vi "thermal_optical_camera_V3.vi"() -> ()   [LabVIEW 2025]
panel:
  in  "File Path":string="C:\\Digambar\\Metal_thin_wall\\Optical_images\\Optical_images"
  in  "Stop (F)":bool
  in  "Acquisition Control:\nExposure Time [100, 3E7]":dbl=999.0 caption="Acquisition Control::Exposure Time" min=100.0 max=29999995.0
  in  "Analog Control:\nGain [0, 27]":dbl caption="Analog Control::Gain" min=0.0 max=27.045663671679687
  in  "Analog Control:\nBlack Level [-5, 10]":dbl caption="Analog Control::Black Level" min=-5.0000011920928955 max=10.000002384185791
  in  "Analog Control:\nGamma [0.25, 4.00]":dbl=0.800048828125 caption="Analog Control::Gamma" min=0.25 max=4.0 step=0.05
  out "Optical camera":T1(plugin-control)
  in  "optical capture interval (s)":dbl
  in  "thermal capture interval (s)":dbl
  out "Thermal camera":T1(plugin-control)
  out "IP address":string
  out "Output":string
  in  "Flag":bool
  in  "Stop recording":bool
  in  "Stop Preview":bool
  in  "Focus":dbl(slide) scale=0.0..100.0
  in  "Record":bool
  out "?":string
  # "Destination for Optical Images:"
  # "change folder name every time you run,\nso it saves each data set in dedicated folder:\nfolder1\nfolder2\nfolder3\netc..."
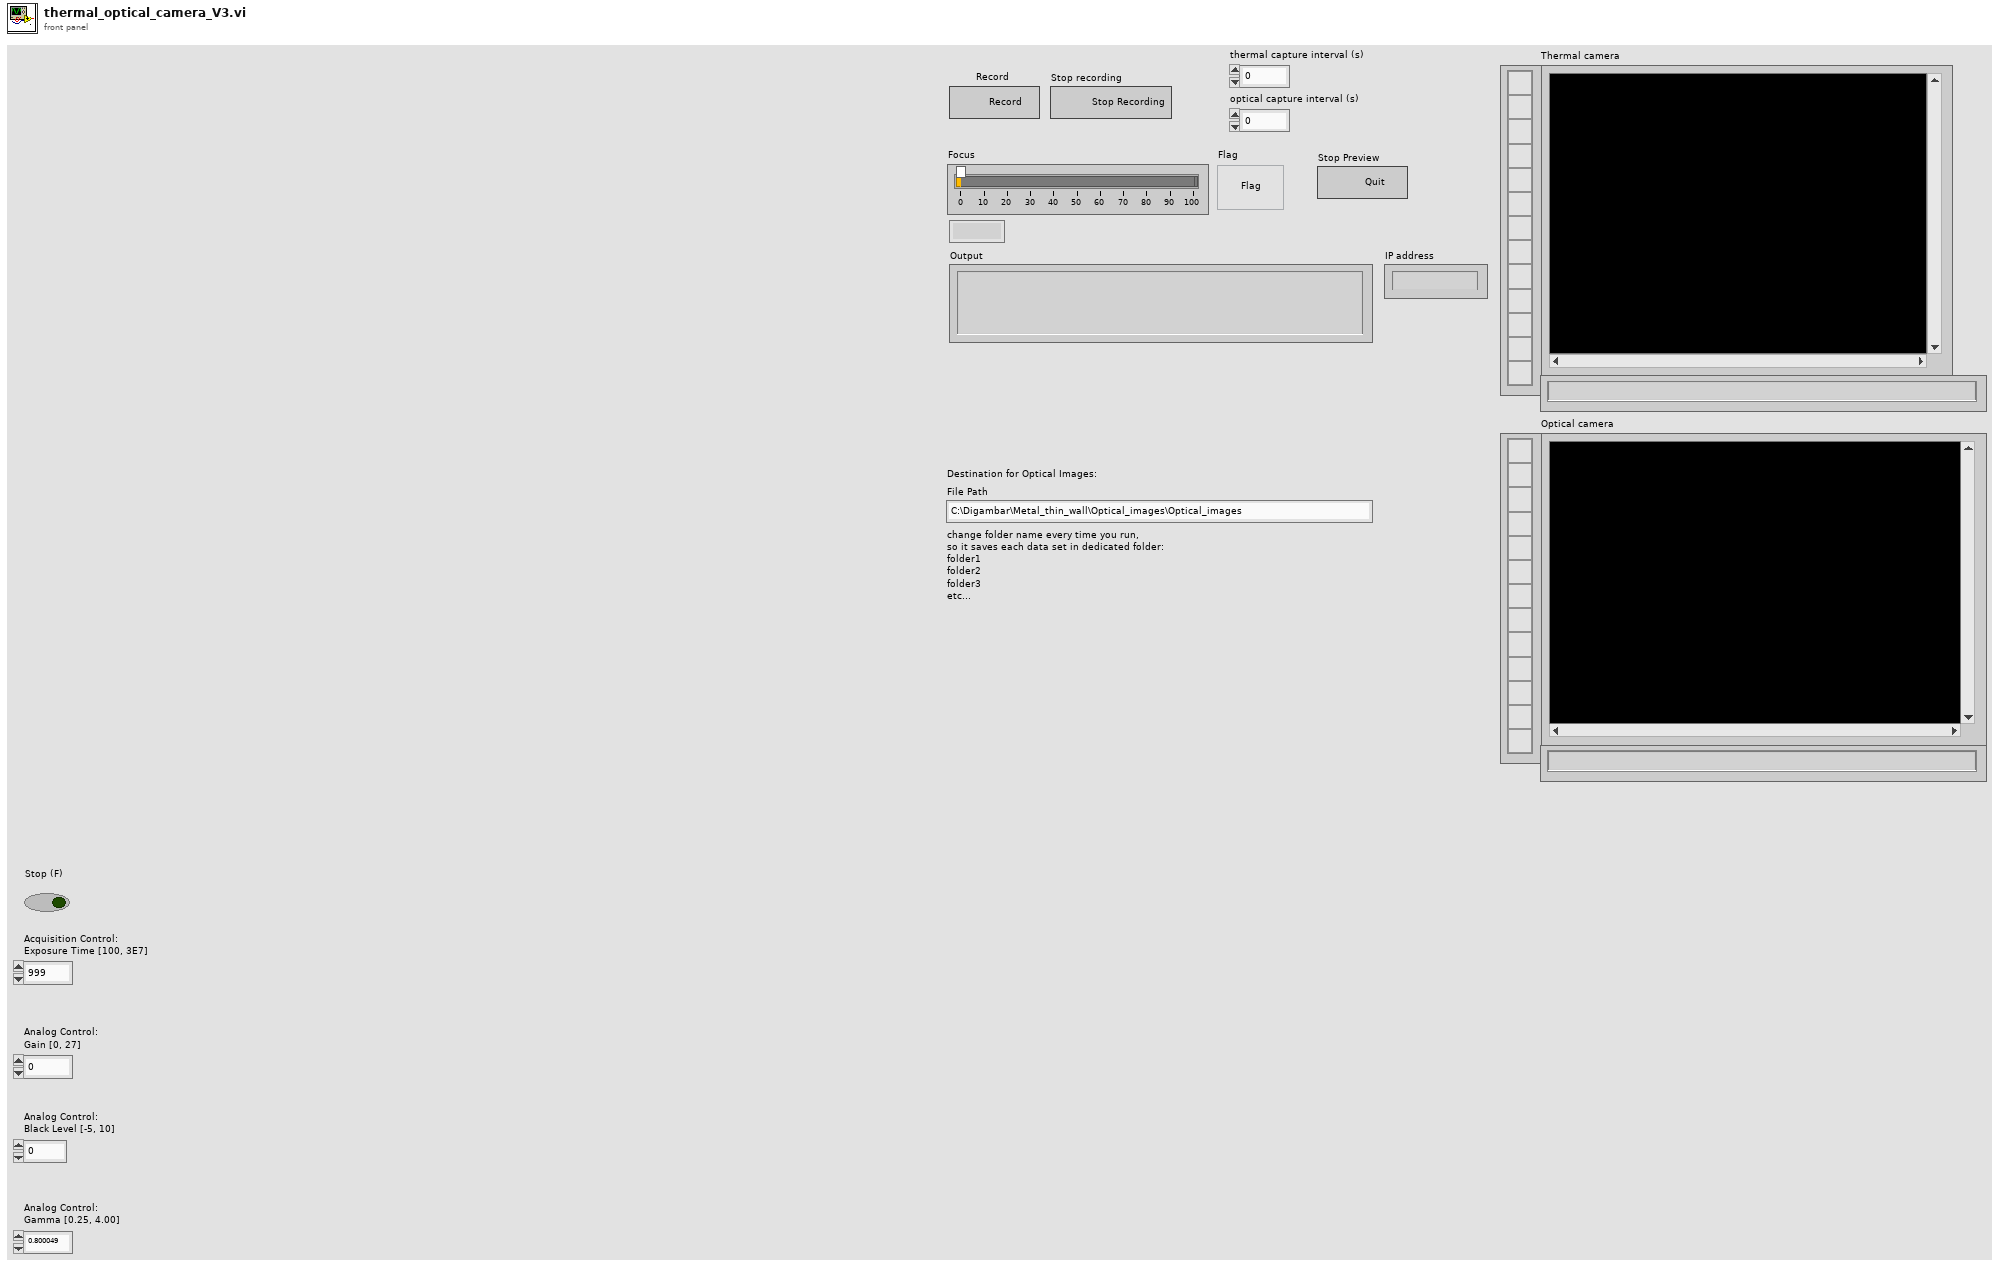
[diagram p1: front panel]
types:
  T1 = typedef "IMAQ Image.ctl" = refnum<image>
  T2 = enum16{"open", "replace", "create", "open or create", "replace or create", "replace or create with confirmation"}
  T3 = enum16{"big-endian, network order", "native, host order", "little-endian"}
  T4 = enum16{"Standard", "Buffered", "CRLF", "Immediate"}
  T5 = typedef "Image Type" = u32
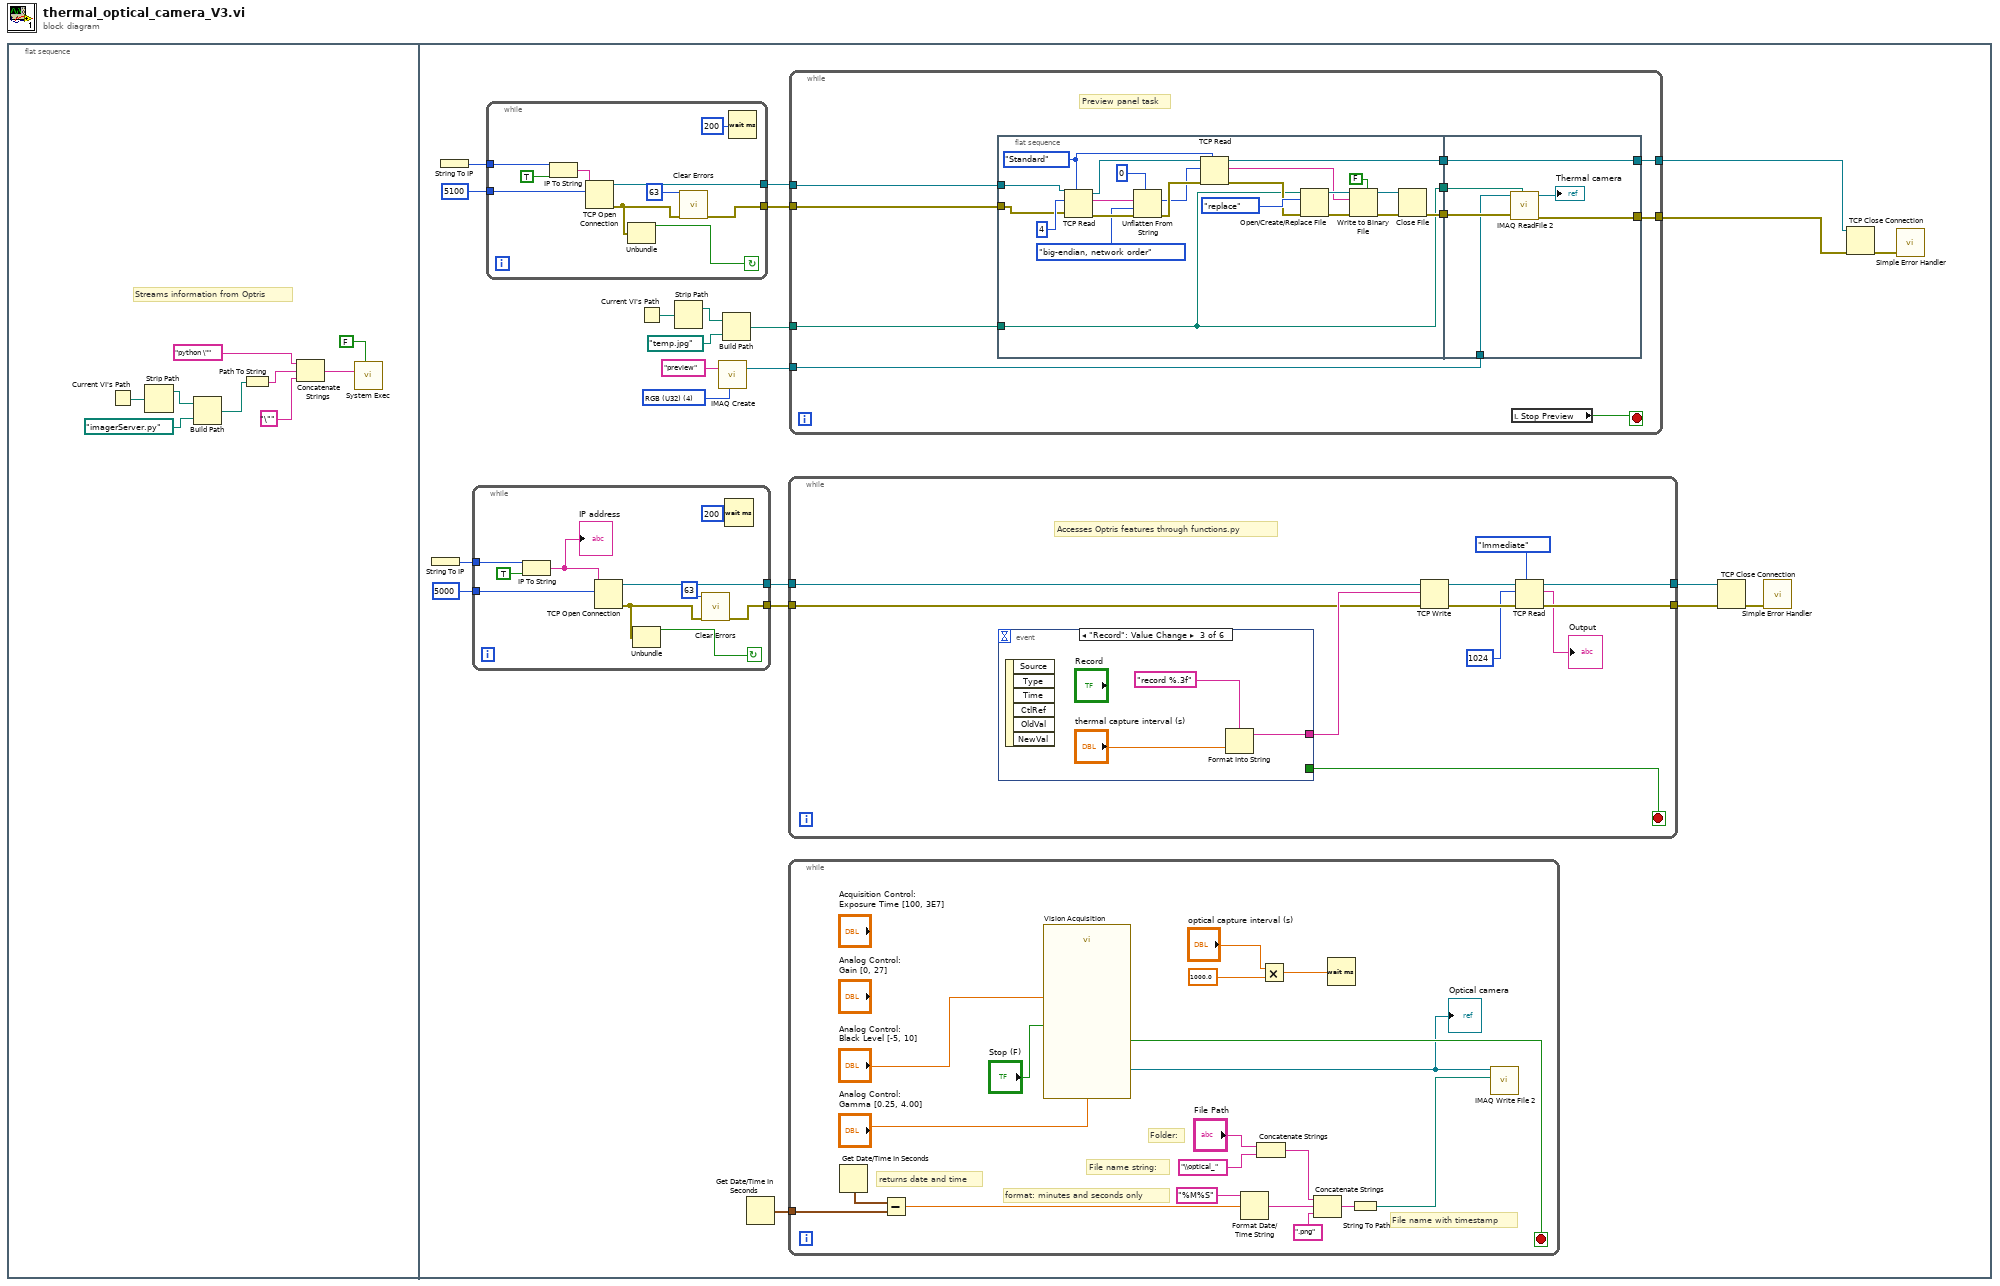
[diagram p0: block diagram]
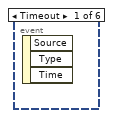
[diagram p2: hidden frame]
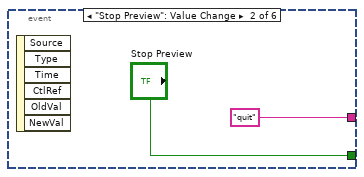
[diagram p3: hidden frame]
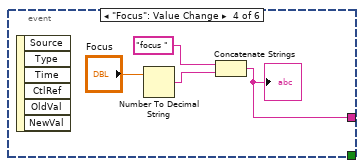
[diagram p4: hidden frame]
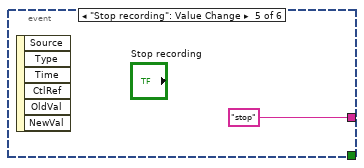
[diagram p5: hidden frame]
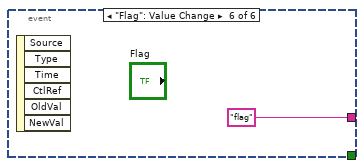
[diagram p6: hidden frame]
diagram:
  n1 = flat-sequence {
    frame #0 {
      # "Streams information from Optris"
      n2 = Current VI's Path() -> (path=w4:path)
      n3 = Strip Path(path=w4) -> (stripped path=w5:path)  [unwired: 1 out]
      n4 = Build Path(base path=w5, name or relative path=path "imagerServer.py") -> (appended path=w2:path)
      n5 = Path To String(path=w2) -> (string=w8:string)
      n6 = Concatenate Strings("python \"" ("string"), w8, "\"" ("string")) -> (w7:string)
      n7 = call <vilib>:"System Exec.vi"("wait until completion? (T)"=FALSE, "command line"=w7) -> ()  [unwired: 6 in, 4 out]
    }
    frame #1 {
      w19 = T5 4 items=["Grayscale (U8)", "Grayscale (I16)", "Grayscale (SGL)", "Complex (CSG)", "RGB (U32)", "HSL (U32)", "RGB (U64)", "Grayscale (U16)"] ("Image Type")
      n8 = String To IP() -> (0:w16:u32)  [unwired: 1 in]
      n9 = String To IP() -> (0:w14:u32)  [unwired: 1 in]
      n10 = while {
        tunnel: [w64] -> w18
        tunnel: [w70] -> w17
        tunnel: w16 -> [w68]
        tunnel: u16 5000 ("remote port or service name") -> [w66]
        stop <- w61 continue-if-true
        n11 = IP To String(1:TRUE ("dot notation? (F)"), 2:w68) -> (0:w69:string)
        "IP address" <- w69
        n12 = TCP Open Connection(address=w69, remote port or service name=w66) -> (connection ID=w70:refnum<k5>, error out=w65:errorcluster)  [unwired: 3 in]
        n13 = Unbundle(w65) -> ("status"=w61:bool)  [unwired: 2 out]
        n14 = call <vilib>:"Clear Errors.vi"("error in (no error)"=w65, "specific error code to clear (0: all)"=63) -> ("error out"=w64:errorcluster)  [unwired: 4 in, 1 out]
        n15 = Wait (ms)(milliseconds to wait=u32 200) -> ()  [unwired: 1 out]
      }
      n16 = while {
        tunnel: w14 -> [w60]
        tunnel: [w54] -> w13
        tunnel: [w58] -> w12
        tunnel: u16 5100 ("remote port or service name") -> [w56]
        stop <- w51 continue-if-true
        n17 = IP To String(1:TRUE ("dot notation? (F)"), 2:w60) -> (0:w59:string)
        n18 = TCP Open Connection(address=w59, remote port or service name=w56) -> (connection ID=w58:refnum<k5>, error out=w55:errorcluster)  [unwired: 3 in]
        n19 = Unbundle(w55) -> ("status"=w51:bool)  [unwired: 2 out]
        n20 = call <vilib>:"Clear Errors.vi"("error in (no error)"=w55, "specific error code to clear (0: all)"=63) -> ("error out"=w54:errorcluster)  [unwired: 4 in, 1 out]
        n21 = Wait (ms)(milliseconds to wait=u32 200) -> ()  [unwired: 1 out]
      }
      n22 = Current VI's Path() -> (path=w30:path)
      n23 = Strip Path(path=w30) -> (stripped path=w31:path)  [unwired: 1 out]
      n24 = call "IMAQ Create"("Image Name"="preview", "Image Type"=w19) -> ("New Image"=w26:T1)  [unwired: 3 in, 1 out]
      n25 = Build Path(base path=w31, name or relative path=path "temp.jpg") -> (appended path=w29:path)
      n26 = Get Date/Time In Seconds() -> (seconds since 1Jan1904=w10:timestamp)
      n27 = while {
        tunnel: [w118] -> w22
        tunnel: [w116] -> w23
        tunnel: w18 -> [w114]
        tunnel: w17 -> [w113]
        stop <- w109 stop-if-true
        # "Accesses Optris features through functions.py"
        n28 = event shown="[2] \"Record\": Value Change" {
          selector: _ -> [_ _ _ _ _ _]
          dyn-events: _ -> [_ _ _ _ _ _]
          timeout: _ -> [_ _ _ _ _ _]
          tunnel: [_ "quit" w124 w126 "stop" "flag"] -> w115
          tunnel: [_ "Stop Preview" _ _ _ _] -> w109
          event Timeout {
            n29 = event-data() -> ()  [unwired: 1 in, 3 out]
          }
          event "Stop Preview": Value Change {
            n30 = event-data() -> ()  [unwired: 1 in, 6 out]
          }
          event "Record": Value Change {
            n31 = event-data() -> ()  [unwired: 1 in, 6 out]
            n32 = Format Into String(format string="record %.3f", "thermal capture interval (s)") -> (resulting string=w124:string)  [unwired: 2 in, 1 out]
          }
          event "Focus": Value Change {
            n33 = event-data() -> ()  [unwired: 1 in, 6 out]
            n34 = Number To Decimal String(number="Focus") -> (decimal integer string=w128:string)  [unwired: 1 in]
            n35 = Concatenate Strings("focus ", w128) -> (w126:string)
            "?" <- w126
          }
          event "Stop recording": Value Change {
            n36 = event-data() -> ()  [unwired: 1 in, 6 out]
          }
          event "Flag": Value Change {
            n37 = event-data() -> ()  [unwired: 1 in, 6 out]
          }
        }
        n38 = TCP Write(connection ID=w113, data in=w115, error in (no error)=w114) -> (connection ID out=w117:refnum<k5>, error out=w119:errorcluster)  [unwired: 1 in, 1 out]
        n39 = TCP Read(connection ID=w117, bytes to read=1024, error in (no error)=w119, 7:T4."Immediate" ("mode (standard)")) -> (connection ID out=w116:refnum<k5>, data out=→"Output":string, error out=w118:errorcluster)  [unwired: 1 in]
      }
      n40 = while {
        tunnel: w10 -> [w36]
        stop <- w49 stop-if-true
        # "format: minutes and seconds only"
        # "returns date and time"
        # "File name with timestamp"
        # "Folder:"
        # "File name string:"
        n41 = Get Date/Time In Seconds() -> (seconds since 1Jan1904=w37:timestamp)
        n42 = Subtract(x=w37, y=w36) -> (x-y=w35:dbl)
        n43 = call "Vision Acquisition"("Analog Control::Black Level"="Analog Control:\nBlack Level [-5, 10]", "Analog Control::Gamma"="Analog Control:\nGamma [0.25, 4.00]", "Stop (F)"="Stop (F)") -> ("Image Out"=w48:T1, "Stopped"=w49:bool)  [unwired: 22 in, 1 out]
        "Optical camera" <- w48
        n44 = Format Date/Time String(time format string (%c)="%M%S", seconds (now)=w35) -> (date/time string=w39:string)  [unwired: 1 in]
        n45 = Concatenate Strings("File Path", "\\optical_" ("string")) -> (w33:string)
        n46 = Multiply(x="optical capture interval (s)", y=1000.0) -> (x*y=w43:dbl)
        n47 = Concatenate Strings(w33, w39, ".png" ("string")) -> (w45:string)
        n48 = Wait (ms)(milliseconds to wait=w43) -> ()  [unwired: 1 out]
        n49 = String To Path(string=w45) -> (path=w41:path)
        n50 = call-poly "IMAQ Write File 2"("File Path"=w41, "Image"=w48) -> ()  [unwired: 8 in, 2 out]
      }
      n51 = while {
        tunnel: w26 -> [w75]
        tunnel: [w76] -> w27
        tunnel: [w80] -> w28
        tunnel: w29 -> [w78]
        tunnel: w13 -> [w73]
        tunnel: w12 -> [w72]
        stop <- w71 stop-if-true
        # "Preview panel task"
        n52 = flat-sequence {
          tunnel: w78 -> [w84]
          tunnel: [w86] -> w79
          tunnel: [w85] -> w77
          tunnel: [w84] -> w74
          tunnel: w73 -> [w82]
          tunnel: w72 -> [w81]
          tunnel: [w108] -> w80
          tunnel: w79 -> [w108]
          tunnel: w77 -> [w107]
          tunnel: [w106] -> w76
          tunnel: w75 -> [w105]
          tunnel: w74 -> [w104]
          frame #0 {
            w95 = T4."Standard" ("mode (standard)")
            n53 = TCP Read(connection ID=w81, bytes to read=4, error in (no error)=w82, 7:w95) -> (connection ID out=w98:refnum<k5>, data out=w83:string, error out=w101:errorcluster)  [unwired: 1 in]
            n54 = Unflatten From String(type=0, binary string=w83, byte order (0:big-endian, network order)=T3."big-endian, network order", error in (no error)=w101) -> (value=w96:i32, error out=w97:errorcluster)  [unwired: 1 in, 1 out]
            n55 = TCP Read(connection ID=w98, bytes to read=w96, error in (no error)=w97, 7:w95) -> (connection ID out=w86:refnum<k5>, data out=w91:string, error out=w93:errorcluster)  [unwired: 1 in]
            n56 = Open/Create/Replace File(file path (use dialog)=w84, error in=w93, operation (0:open)=T2."replace") -> (refnum out=w92:refnum<file>, error out=w89:errorcluster)  [unwired: 3 in, 1 out]
            n57 = Write to Binary File(file (use dialog)=w92, data=w91, error in=w89, 5:FALSE ("prepend array or string size? (T)")) -> (refnum out=w87:refnum<file>, error out=w88:errorcluster)  [unwired: 2 in, 1 out]
            n58 = Close File(refnum=w87, error in=w88) -> (error out=w85:errorcluster)  [unwired: 1 out]
          }
          frame #1 {
            n59 = call "IMAQ ReadFile 2"("File Path"=w104, "error in (no error)"=w107, "Image"=w105) -> ("error out"=w106:errorcluster, "Image Out"=→"Thermal camera":T1)  [unwired: 4 in, 3 out]
          }
        }
        n60 = local read "Stop Preview"() -> (w71:bool)
      }
      n61 = TCP Close Connection(connection ID=w23, error in (no error)=w22) -> (error out=w24:errorcluster)  [unwired: 1 in, 1 out]
      n62 = call <vilib>:"Simple Error Handler.vi"("error in (no error)"=w24) -> ()  [unwired: 4 in, 5 out]
      n63 = TCP Close Connection(connection ID=w28, error in (no error)=w27) -> (error out=w25:errorcluster)  [unwired: 1 in, 1 out]
      n64 = call <vilib>:"Simple Error Handler.vi"("error in (no error)"=w25) -> ()  [unwired: 4 in, 5 out]
    }
  }
